vi "ClsOpenConnection.vi"(6 "error in":errorcluster, 8 "Device Type":i32, 9 "Connection Info":string) -> (0 "error out":errorcluster, 3 "Connection Handle out":u32)   [LabVIEW 2015]
doc: "Open Connection:\n\nYou must use this vi to connect to the device before any other functions are used.\n\nConnection Info[Input]: is like \"COM 15\" for serial connection and \"IP: 192.168.170.2\" for ethernet connection.\n\nDevice Type[Input]: 0 for first generation CHRocodile devices; 1 for CHRocodile 2 devices; 2 for CLS/MPS devices.\n\nConnection Handle Out[Output]: the created connection handle. Refer to this handle when you refer to the same connection."
uses:
  W:/Drop Impact Teststand/dependent dlls/CHRocodileDLL.dll
panel:
  in  "Handle":u32
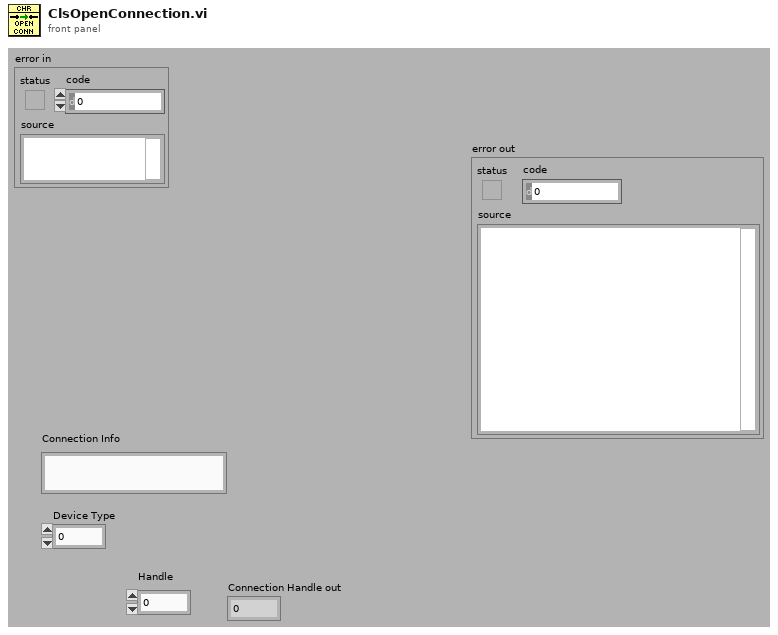
[diagram p1: front panel]
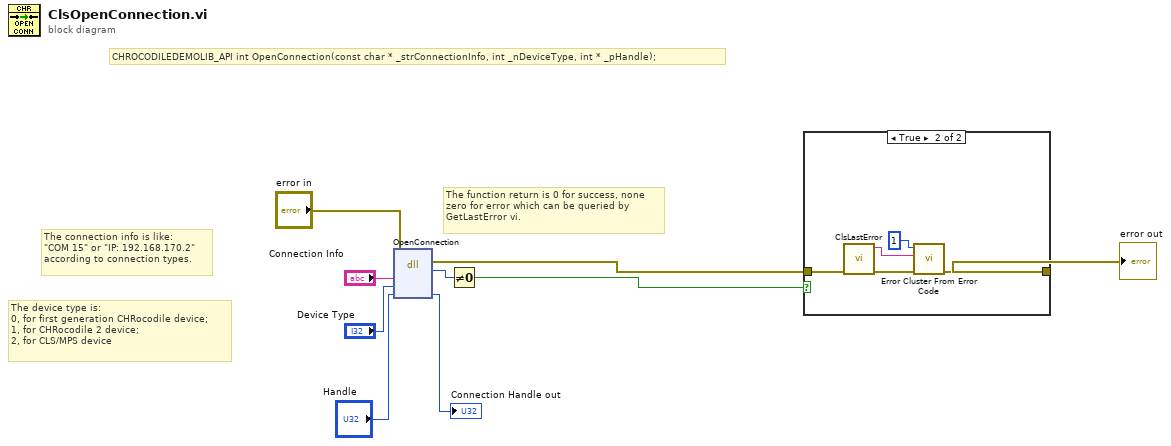
[diagram p0: block diagram]
diagram:
  # "The function return is 0 for success, none\nzero for error which can be queried by\nGetLastError vi."
  # "The device type is:\n0, for first generation CHRocodile device; \n1, for CHRocodile 2 device; \n2, for CLS/MPS device"
  # "The connection info is like:\n\"COM 15\" or \"IP: 192.168.170.2\"\naccording to connection types."
  # "CHROCODILEDEMOLIB_API int OpenConnection(const char * _strConnectionInfo, int _nDeviceType, int * _pHandle);"
  n1 = dll-call lib="W:/Drop Impact Teststand/dependent dlls/CHRocodileDLL.dll" fn="OpenConnection"(error in="error in", "_strConnectionInfo"="Connection Info", "_nDeviceType"="Device Type", "_pHandle"="Handle") -> (error out=w3:errorcluster, "return"=w5:i32, "_pHandle"=→"Connection Handle out":u32)  [unwired: 4 in, 1 out]
  n2 = Not Equal To 0?(x=w5) -> (x != 0?=w4:bool)
  n3 = case shown="True" w4 {
    tunnel: [w10 w11] -> w1
    tunnel: w3 -> [w10 w14]
    frame False {
    }
    frame True {
      n4 = call "ClsLastError.vi"("error in (no error)"=w14) -> ("error out"=w13:errorcluster, "Error Message"=w12:string)  [unwired: 9 in]
      n5 = call <vilib>:"Error Cluster From Error Code.vi"("error in (no error)"=w13, "error message (\"\")"=w12, "error code (0)"=1) -> ("error out"=w11:errorcluster)  [unwired: 6 in]
    }
  }
  "error out" <- w1
